vi "Get DLL Path.vi"() -> (0 "DLL Path":path)   [LabVIEW 2024, in "Keyence LK-G3000.lvlib"]
uses:
  Keyence LK-G3000.lvlib
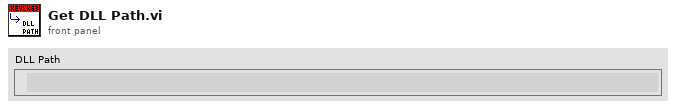
[diagram p1: front panel]
types:
  T1 = enum32{"invalid app kind", "Development System", "Run Time System", "Student Edition", "Embedded LabVIEW", "Evaluation", "Custom"}
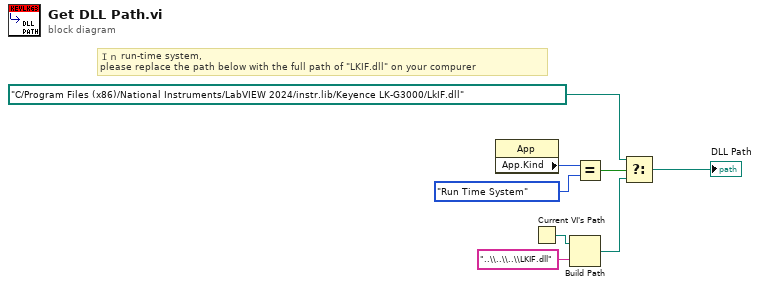
[diagram p0: block diagram]
diagram:
  # "Ｉｎ run-time system,\nplease replace the path below with the full path of \"LKIF.dll\" on your compurer"
  n1 = property class="App"() -> ("App.Kind"=w8:T1)  [unwired: 2 in, 2 out]
  n2 = Current VI's Path() -> (path=w5:path)
  n3 = Build Path(base path=w5, name or relative path="..\\..\\..\\LKIF.dll" ("名前または相対パス")) -> (appended path=w3:path)
  n4 = Equal?(x=w8, y=T1."Run Time System") -> (x = y?=w6:bool)
  n5 = Select(t=path "C:/Program Files (x86)/National Instruments/LabVIEW 2024/instr.lib/Keyence LK-G3000/LkIF.dll", s=w6, f=w3) -> (s? t:f=→"DLL Path":path)
